vi "C37 Get PMU Data.vi"(7 "Channel Info":T2, 8 "error in (no error)":errorcluster, 10 "PMU Index":i32, 11 "Pseudo PDC ID":i32) -> (0 "error out":errorcluster, 1 "Digital Values":bool[](array[boolean]), 2 "Analog Values":sgl[](array[numeric]), 3 "Phasor Values":csg[](array[numeric]), 4 "Frequency":sgl, 5 "status":T1, 6 "Delta Frequency":sgl)   [LabVIEW 2013, in "C37118-DLL.lvlib"]
uses:
  C37118-DLL.lvlib
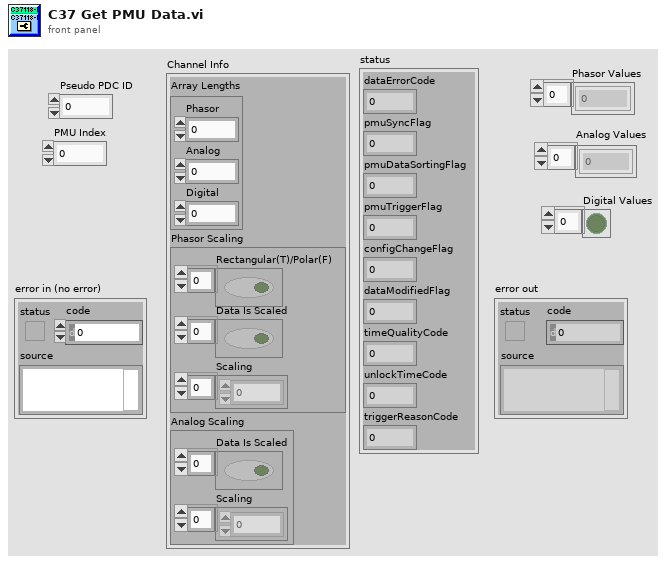
[diagram p1: front panel]
types:
  T1 = cluster{"dataErrorCode":u8, "pmuSyncFlag":u8, "pmuDataSortingFlag":u8, "pmuTriggerFlag":u8, "configChangeFlag":u8, "dataModifiedFlag":u8, "timeQualityCode":u8, "unlockTimeCode":u8, "triggerReasonCode":u8}
  T2 = cluster{"Array Lengths":cluster{"Phasor":i32, "Analog":i32, "Digital":i32}, "Phasor Scaling":cluster{"Rectangular(T)/Polar(F)":bool[], "Data Is Scaled":bool[], "Scaling":sgl[]}, "Analog Scaling":cluster{"Data Is Scaled":bool[], "Scaling":sgl[]}}
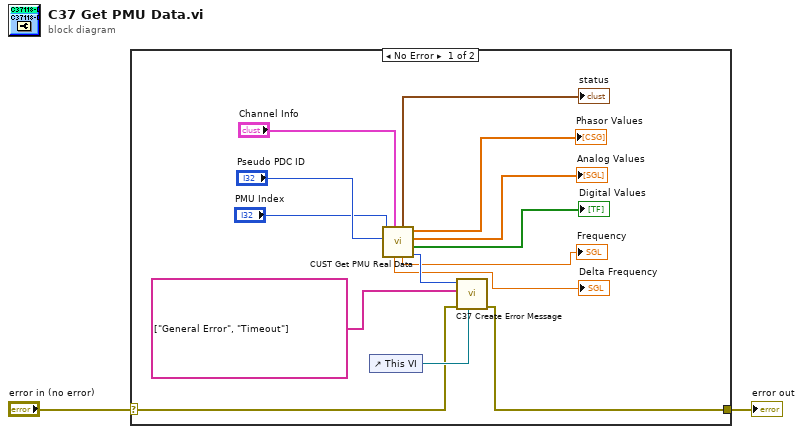
[diagram p0: block diagram]
diagram:
  n1 = case shown="No Error" "error in (no error)" {
    selector: "error in (no error)" -> [w15 w17]
    tunnel: [w14 w17] -> w2
    frame No Error {
      n2 = control-ref of="This VI"() -> (w16:refnum<vi>)
      n3 = call "CUST Get PMU Real Data.vi"("Channel Info"="Channel Info", "pseudoPdcId"="Pseudo PDC ID", "pmuIndex"="PMU Index") -> ("function return"=w10:i32, "Digital Values"=→"Digital Values":bool[], "Analog Values"=→"Analog Values":sgl[], "Phasor Values"=→"Phasor Values":csg[], "Frequency"=→"Frequency":sgl, "status"=→"status":T1, "Delta Frequency"=→"Delta Frequency":sgl)  [unwired: 2 in]
      n4 = call "C37 Create Error Message.vi"("VI Reference"=w16, "error in (no error)"=w15, "Error Messages"=string[] ["General Error", "Timeout"], "function return"=w10) -> ("error out"=w14:errorcluster)  [unwired: 7 in]
    }
    frame Error {
    }
  }
  "error out" <- w2
